vi "Cursors Snap Query.vi"(8 "error in":errorcluster, 11 "Instrument Handle In":i32) -> (0 "error out":errorcluster, 2 "State":i32, 3 "Instrument Handle Out":i32)   [LabVIEW 8.6, in "ZTScopeM.lvlib"]
doc: "Query the state of the cursors snap to waveform."
uses:
  ZTScopeM.lvlib
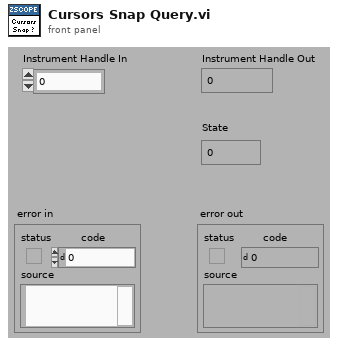
[diagram p1: front panel]
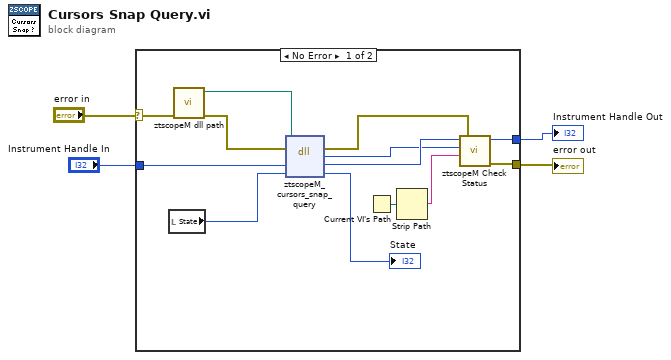
[diagram p0: block diagram]
diagram:
  n1 = case shown="No Error" "error in" {
    selector: "error in" -> [w8 w19]
    tunnel: [w11 w19] -> w1
    tunnel: "Instrument Handle In" -> [w17 w18]
    tunnel: [w12 w18] -> w3
    frame #0 {
      n2 = local read "State"() -> (w10:i32)
      n3 = call "ztscopeM dll path.vi"("error in (no error)"=w8) -> ("error out"=w6:errorcluster, "<instrument>.dll path"=w7:path)  [unwired: 9 in]
      n4 = dll-call lib="C:/Program Files (x86)/National Instruments/LabVIEW 2013/instr.lib/ztscopem/ztscopeM.dll" fn="ztscopeM_cursors_snap_query"(path in=w7, error in=w6, "instrumentHandle"=w17, "state"=w10) -> (error out=w5:errorcluster, w13:i32, "instrumentHandle"=w14:i32, "state"=→"State":i32)  [unwired: 1 in, 1 out]
      n5 = Current VI's Path() -> (path=w16:path)
      n6 = Strip Path(path=w16) -> (name=w15:string)  [unwired: 1 out]
      n7 = call "ztscopeM Check Status.vi"("error in"=w5, "name of VI"=w15, "status (return code)"=w13, "instrument handle in"=w14) -> ("error out"=w11:errorcluster, "instrument handle out"=w12:i32)  [unwired: 2 in]
    }
    frame #1 {
    }
  }
  "Instrument Handle Out" <- w3
  "error out" <- w1
